vi "CRYItems Sort.vi"(9 "Check In":bool[](array[boolean]), 10 "Items In":string[](array[string])) -> (0 "Check Out":bool[](array[boolean]), 2 "Items Out":string[](array[string]))   [LabVIEW 2013]
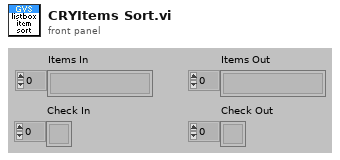
[diagram p1: front panel]
types:
  T1 = cluster{dbl, dbl, "String":string, "Boolean":bool}
  T2 = cluster{dbl, dbl, "String":string, "Boolean":bool}[]
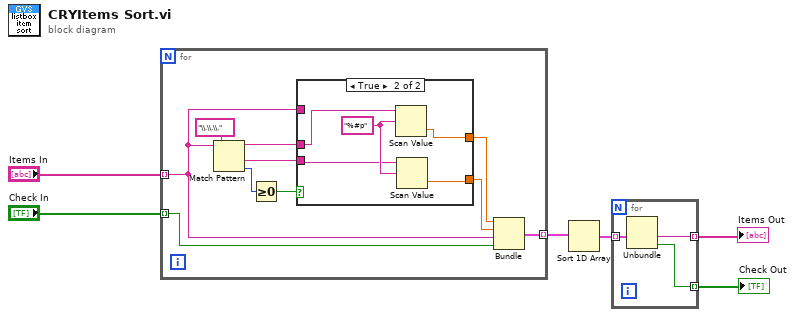
[diagram p0: block diagram]
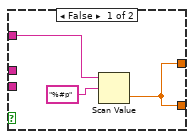
[diagram p2: hidden frame]
diagram:
  n1 = for {
    tunnel: "Items In" -> [w13] mode=indexing
    tunnel: "Check In" -> [w12] mode=indexing
    tunnel: [w11] -> w1 mode=indexing
    n2 = Match Pattern(string=w13, regular expression="\\.\\.\\.") -> (before substring=w10:string, after substring=w9:string, offset past match=w16:i32)  [unwired: 2 out]
    n3 = Greater Or Equal To 0?(x=w16) -> (x >= 0?=w15:bool)
    n4 = case shown="True" w15 {
      tunnel: w13 -> [w19 _]
      tunnel: [w17 w21] -> w8
      tunnel: w10 -> [_ w23]
      tunnel: w9 -> [_ w22]
      tunnel: [w17 w20] -> w7
      frame False {
        n5 = Scan Value(string=w19, format string="%#p") -> (value=w17:dbl)  [unwired: 1 in, 1 out]
      }
      frame True {
        w24 = "%#p" ("format string")
        n6 = Scan Value(string=w23, format string=w24) -> (value=w21:dbl)  [unwired: 1 in, 1 out]
        n7 = Scan Value(string=w22, format string=w24) -> (value=w20:dbl)  [unwired: 1 in, 1 out]
      }
    }
    n8 = Bundle(w8, w7, "String"=w13, "Boolean"=w12) -> (w11:T1)  [unwired: 1 out]
  }
  n9 = Sort 1D Array(array=w1) -> (sorted array=w2:T2)
  n10 = for {
    tunnel: w2 -> [w27] mode=indexing
    tunnel: [w26] -> w3 mode=indexing
    tunnel: [w25] -> w4 mode=indexing
    n11 = Unbundle(w27) -> ("String"=w26:string, "Boolean"=w25:bool)  [unwired: 2 out]
  }
  "Items Out" <- w3
  "Check Out" <- w4
